vi "Read configuration.vi"(8 "error in":errorcluster, 11 "FPGA Module editor node in":refnum<class "FPGA Module editor node.lvclass">) -> (0 "error out":errorcluster, 2 "configuration":refnum<class "NISE_CEF_serializable configuration.lvclass">, 3 "FPGA Module editor node out":refnum<class "FPGA Module editor node.lvclass">)   [LabVIEW 2013, in "FPGA Module editor node.lvclass"]
uses:
  FPGA Module editor node.lvclass
  <vilib>/NI/Configuration Framework/serializable configuration/NISE_CEF_serializable configuration.lvclass
  FPGA Module editor node.lvclass/FPGA Module editor node.ctl
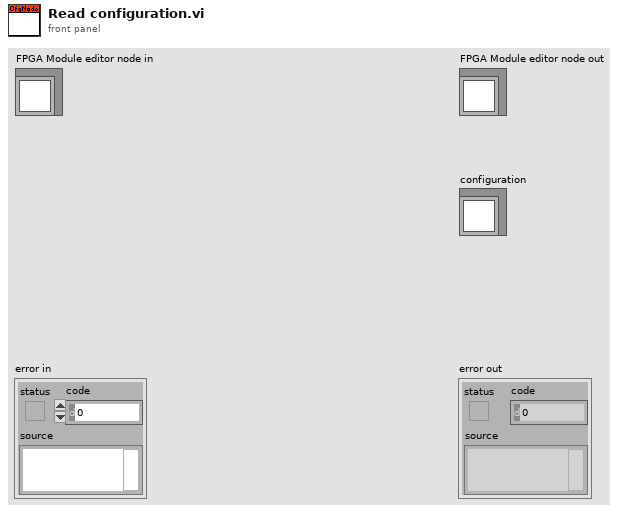
[diagram p1: front panel]
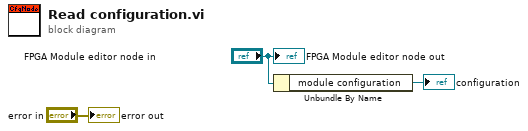
[diagram p0: block diagram]
diagram:
  n1 = Unbundle By Name("FPGA Module editor node in") -> ("module configuration"=→"configuration":refnum<class "FPGA Module configuration.lvclass">)
  "error out" <- "error in"
  "FPGA Module editor node out" <- "FPGA Module editor node in"
